vi "SPC_get_actual_coltime.vi"(8 "Error In":errorcluster, 10 "Module No":i16 min=0 max=7 step=1, 11 "DLL Path":path) -> (0 "Error Out":errorcluster, 2 "Module No":i16 min=0 max=7 step=1, 3 "DLL Path":path, 4 "coltime":sgl format="%.2f")   [LabVIEW 2017]
doc: "The procedure reads the timer for the collection time and calculates the actual collection time value for the SPC module ‘mod_no’. During the measurement this value decreases from the specified collection time to 0.\nFor collection times longer than 80 seconds be sure that SPC_test_state is called in the loop during the measurement before the SPC_get_actual_coltime call. SPC_test_state updates software counter which is needed for times longer than 80 sec.\nIn comparison to the procedure SPC_get_time_from_start, which delivers the real time from start, the procedure returns the actual state of the dead time compensated collection time. At high count rates the real time of collection can be considerably longer than the specified collection time value.\nFor SPC6x0,130 modules only:\n- If the sequencer is running, the collection timer cannot be accessed.\n- The dead time compensation can be switched off. In this case the collection timer runs with the same speed as the repeat timer, and the result is the same as that of the procedure SPC_get_time_from_start."
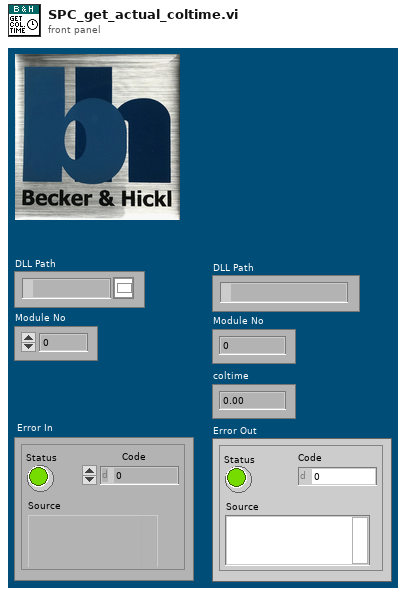
[diagram p1: front panel]
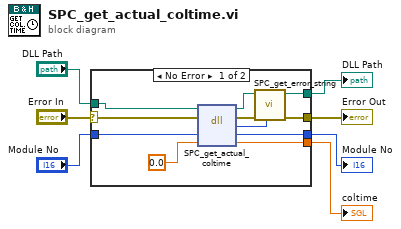
[diagram p0: block diagram]
diagram:
  n1 = case shown="No Error" "Error In" {
    selector: "Error In" -> [w17 w21]
    tunnel: [w13 w20] -> w7
    tunnel: [w14 w21] -> w6
    tunnel: "DLL Path" -> [w18 w20]
    tunnel: "Module No" -> [w11 w19]
    tunnel: [w10 w19] -> w2
    tunnel: [w9 _] -> w1
    frame No Error {
      n2 = dll-call lib="D:/spcm/lib/lab_view/lv10.0/spcm32.dll" fn="SPC_get_actual_coltime"(path in=w18, error in=w17, "mod_no"=w11, "time"=sgl 0.0 ("Last Time Value")) -> (path out=w12:path, error out=w15:errorcluster, "return type"=w16:i16, "mod_no"=w10:i16, "time"=w9:sgl)  [unwired: 1 in]
      n3 = call "SPC_get_error_string.vi"("ErrorID"=w16, "Error In"=w15, "DLL Path"=w12) -> ("Error Out"=w14:errorcluster, "DLL Path"=w13:path)  [unwired: 6 in, 1 out]
    }
    frame Error {
    }
  }
  "DLL Path" <- w7
  "Error Out" <- w6
  "Module No" <- w2
  "coltime" <- w1
